vi "GetCustomElement.vi"(8 "error in":errorcluster, 11 "CustomDataType in":refnum<class "CustomData.lvclass">) -> (0 "error out":errorcluster, 2 "CustomElements":refnum<class "CustomElement.lvclass">[](array[class]), 3 "CustomDataType out":refnum<class "CustomData.lvclass">)   [LabVIEW 2021, in "ProligentXMLGenerator.lvlib" / "CustomData.lvclass"]
doc: "Get CustomElement."
uses:
  CustomData.lvclass
  CustomData.lvclass/CustomData.ctl
  CustomElement/CustomElement.lvclass
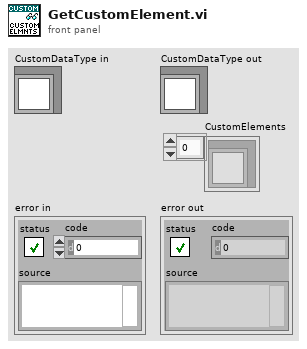
[diagram p1: front panel]
types:
  T1 = typedef "ProligentXMLGenerator.lvlib/CustomData.lvclass/Data.ctl" = cluster{"Name":string, "CustomElements":refnum<class "CustomElement.lvclass">[]}
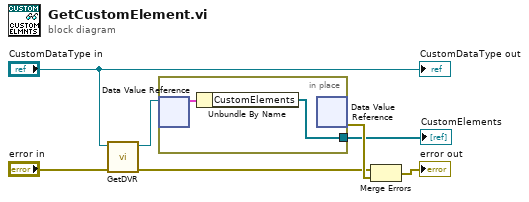
[diagram p0: block diagram]
diagram:
  n1 = call "GetDVR.vi"("error in"="error in", "CustomDataType"="CustomDataType in") -> ("error out"=w1:errorcluster, "DVRReference"=w6:refnum<data-value>)  [unwired: 8 in]
  n2 = in-place "In Place Element Structure" {
    in-place-border: [w8] -> w2
    n3 = in-place-dvr #1(w6) -> (w9:T1)  [unwired: 1 out]
    n4 = Unbundle By Name(w9) -> ("CustomElements"=w8:refnum<class "CustomElement.lvclass">[])
    n5 = in-place-dvr #1() -> (w7:errorcluster)  [unwired: 1 in, 1 out]
  }
  "CustomElements" <- w2
  n6 = Merge Errors(w1, w7) -> (→"error out":errorcluster)
  "CustomDataType out" <- "CustomDataType in"
